vi "Write Output Channels[].vi"(8 "error in (no error)":errorcluster, 10 "Output Channels[]":refnum<class "Output Channels.lvclass">[](array[class]), 11 "Plugin_UI in":refnum<class "Plugin_UI.lvclass">) -> (0 "error out":errorcluster, 3 "Plugin_UI out":refnum<class "Plugin_UI.lvclass">)   [LabVIEW 2020, in "Plugin.lvlib" / "Plugin_UI.lvclass"]
doc: "Writes output channels"
uses:
  Plugin_UI.lvclass
  Channels/Output Channels/Output Channels.lvclass
  Plugin_UI.lvclass/Plugin_UI.ctl
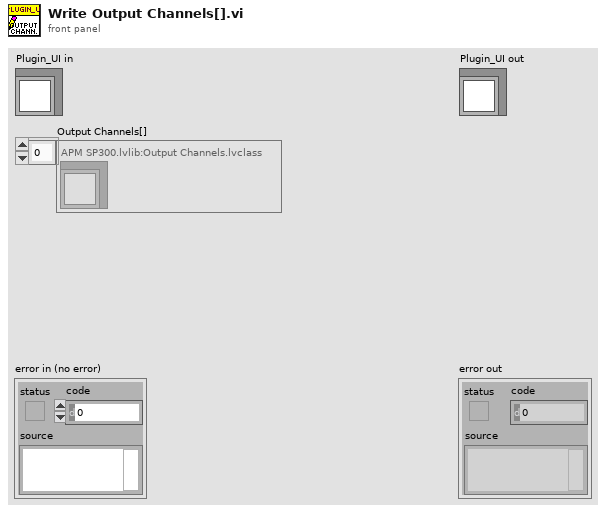
[diagram p1: front panel]
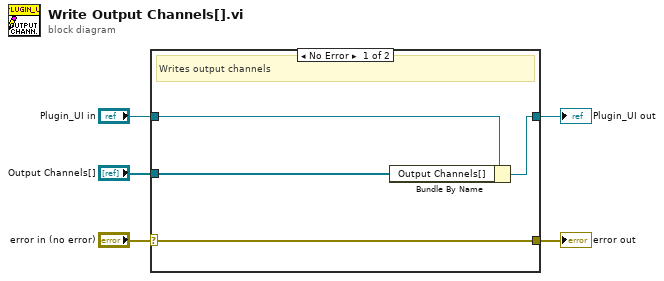
[diagram p0: block diagram]
diagram:
  n1 = case shown="No Error" "error in (no error)" {
    selector: "error in (no error)" -> [w9 w10]
    tunnel: [w9 w10] -> w4
    tunnel: [w7 w11] -> w2
    tunnel: "Plugin_UI in" -> [w8 w11]
    tunnel: "Output Channels[]" -> [w6 _]
    frame No Error {
      # "Writes output channels"
      n2 = Bundle By Name(cluster=w8, "Output Channels[]"=w6) -> (w7:refnum<class "Plugin_UI.lvclass">)
    }
    frame Error {
    }
  }
  "error out" <- w4
  "Plugin_UI out" <- w2
